vi "CLI_ParseParam.vi"(8 "error in (no error)":errorcluster caption="entrée d'erreur (pas d'erreur)") -> (0 "Error out":errorcluster, 1 "ParsedParameters":cluster{"Name":string, "Value":string}[](array[cluster]), 2 "Is_RunTime":bool, 3 "CliParametres":string[](array[string]))   [LabVIEW 2013]
panel:
  in  "Bouton Stop":bool
  in  "Ref_Launcher":refnum<vi>
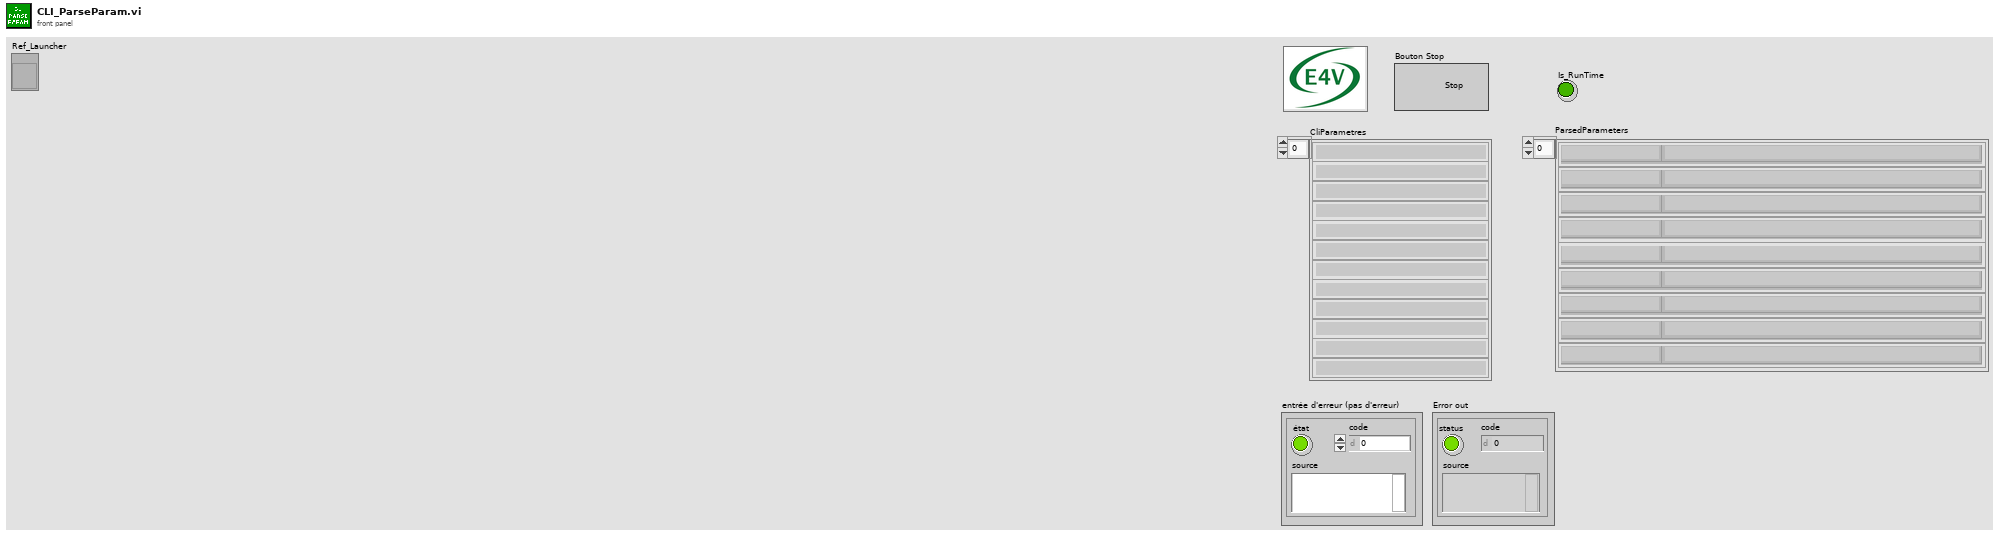
[diagram p1: front panel]
types:
  T1 = enum32{"invalid app kind", "Development System", "Run Time System", "Student Edition", "Embedded LabVIEW", "Evaluation", "Custom"}
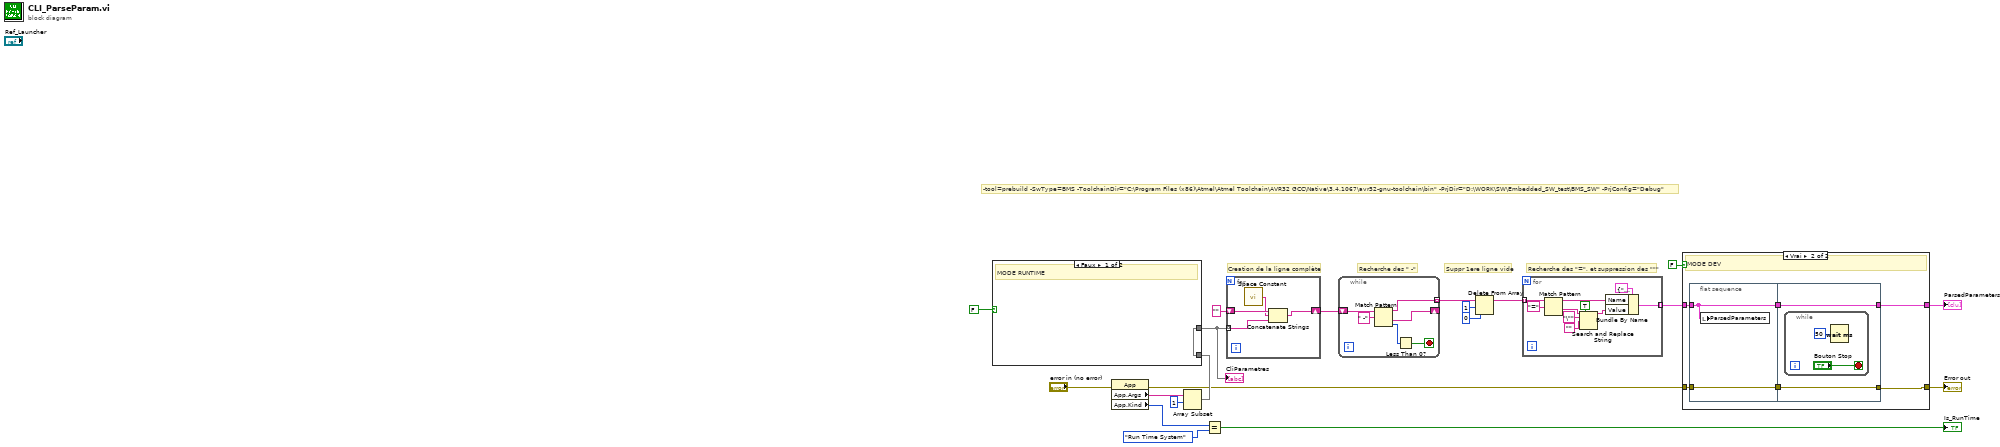
[diagram p0: block diagram]
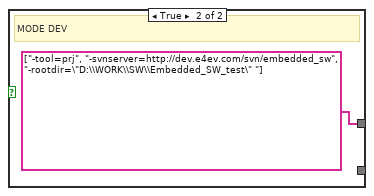
[diagram p3: hidden frame]
diagram:
  # "-tool=prebuild -SwType=BMS -ToolchainDir=\"C:\\Program Files (x86)\\Atmel\\Atmel Toolchain\\AVR32 GCC\\Native\\3.4.1067\\avr32-gnu-toolchain\\bin\" -PrjDir=\"D:\\WORK\\SW\\Embedded_SW_test\\BMS_SW\" -PrjConfig=\"Debug\""
  # "Suppr 1ere ligne vide"
  # "Recherche des \"=\", et suppression des \"\"\""
  # "Recherche des \" -\""
  # "Creation de la ligne complète"
  n1 = property class="App"(error in="error in (no error)") -> (error out=w6:errorcluster, "App.Args"=w19:string[], "App.Kind"=w17:T1)  [unwired: 1 in, 1 out]
  n2 = Array Subset(array=w19, index=1 ("indice")) -> (w11:string[])  [unwired: 1 in]
  n3 = case shown="Faux" FALSE {
    tunnel: w11 -> [w21 _]
    tunnel: [w21 string[] ["-tool=prj", "-svnserver=http://dev.e4ev.com/svn/embedded_sw", "-rootdir=\"D:\\WORK\\SW\\Embedded_SW_test\" "]] -> w2
    frame False {
      # "MODE RUNTIME"
    }
    frame True {
      # "MODE DEV"
    }
  }
  "CliParametres" <- w2
  n4 = Equal?(x=w17, y=T1."Run Time System" ("Application:Type")) -> (x = y?=→"Is_RunTime":bool)
  n5 = for {
    tunnel: w2 -> [w24] mode=indexing
    shift-right: [w25] -> w3
    shift-left: "" -> [w26]
    n6 = call <vilib>:"Space Constant.vi"() -> ("String"=w23:string)
    n7 = Concatenate Strings(w26, w23, w24) -> (w25:string)
  }
  n8 = while {
    shift-right: [w29] -> _
    shift-left: w3 -> [w31]
    tunnel: [w28] -> w15 mode=indexing
    stop <- w30 stop-if-true
    n9 = Match Pattern(string=w31, regular expression=" -" ("expression régulière")) -> (before substring=w28:string, after substring=w29:string, offset past match=w27:i32)  [unwired: 1 in, 1 out]
    n10 = Less Than 0?(x=w27) -> (x < 0?=w30:bool)
  }
  n11 = Delete From Array(array=w15, length=1 ("longueur"), index=0 ("indice")) -> (array with subset deleted=w12:string[])  [unwired: 1 out]
  n12 = for {
    tunnel: w12 -> [w33] mode=indexing
    tunnel: [w39] -> w9 mode=indexing
    n13 = Match Pattern(string=w33, regular expression="=" ("expression régulière")) -> (before substring=w40:string, after substring=w37:string)  [unwired: 1 in, 2 out]
    n14 = Search and Replace String(replace all?=TRUE ("tout remplacer ? (F)"), input string=w37, search string="\"" ("chaîne recherchée"), replace string="") -> (result string=w34:string)  [unwired: 4 in, 3 out]
    n15 = Bundle By Name(cluster=cluster{"Name":string, "Value":string} {"Name"="", "Value"=""} ("ParsedParameter"), "Name"=w40, "Value"=w34) -> (w39:cluster{"Name":string, "Value":string})
  }
  n16 = case shown="Vrai" FALSE {
    tunnel: [w44 w45] -> w8
    tunnel: w9 -> [w44 w50]
    tunnel: [w43 w47] -> w7
    tunnel: w6 -> [w43 w49]
    frame False {
      # "MODE NORMAL"
    }
    frame True {
      # "MODE DEV"
      n17 = flat-sequence {
        tunnel: w50 -> [w51]
        tunnel: w49 -> [w52]
        tunnel: [w52] -> w48
        tunnel: [w51] -> w46
        tunnel: [w54] -> w47
        tunnel: w48 -> [w54]
        tunnel: [w53] -> w45
        tunnel: w46 -> [w53]
        frame #0 {
          n18 = local write "ParsedParameters"(w51) -> ()
        }
        frame #1 {
          n19 = while {
            stop <- "Bouton Stop" stop-if-true
            n20 = Wait (ms)(milliseconds to wait=u32 50 ("attente (ms)")) -> ()  [unwired: 1 out]
          }
        }
      }
    }
  }
  "Error out" <- w7
  "ParsedParameters" <- w8
